vi "TDMSVisuSimple.vi"(4 "entrée d'erreur":errorcluster caption="entrée d'erreur (pas d'erreur)", 7 "chemin du fichier":path) -> (0 "sortie d'erreur":errorcluster)   [LabVIEW 2017]
panel:
  out "FileInfo":string
  out "Chaîne":string
  in  "RemoveAll":bool
  in  "DisplayAll":bool
  in  "Quitter":bool
  out "Graphe":waveform(dbl)[](graph)
  # "File information"
  # "Data"
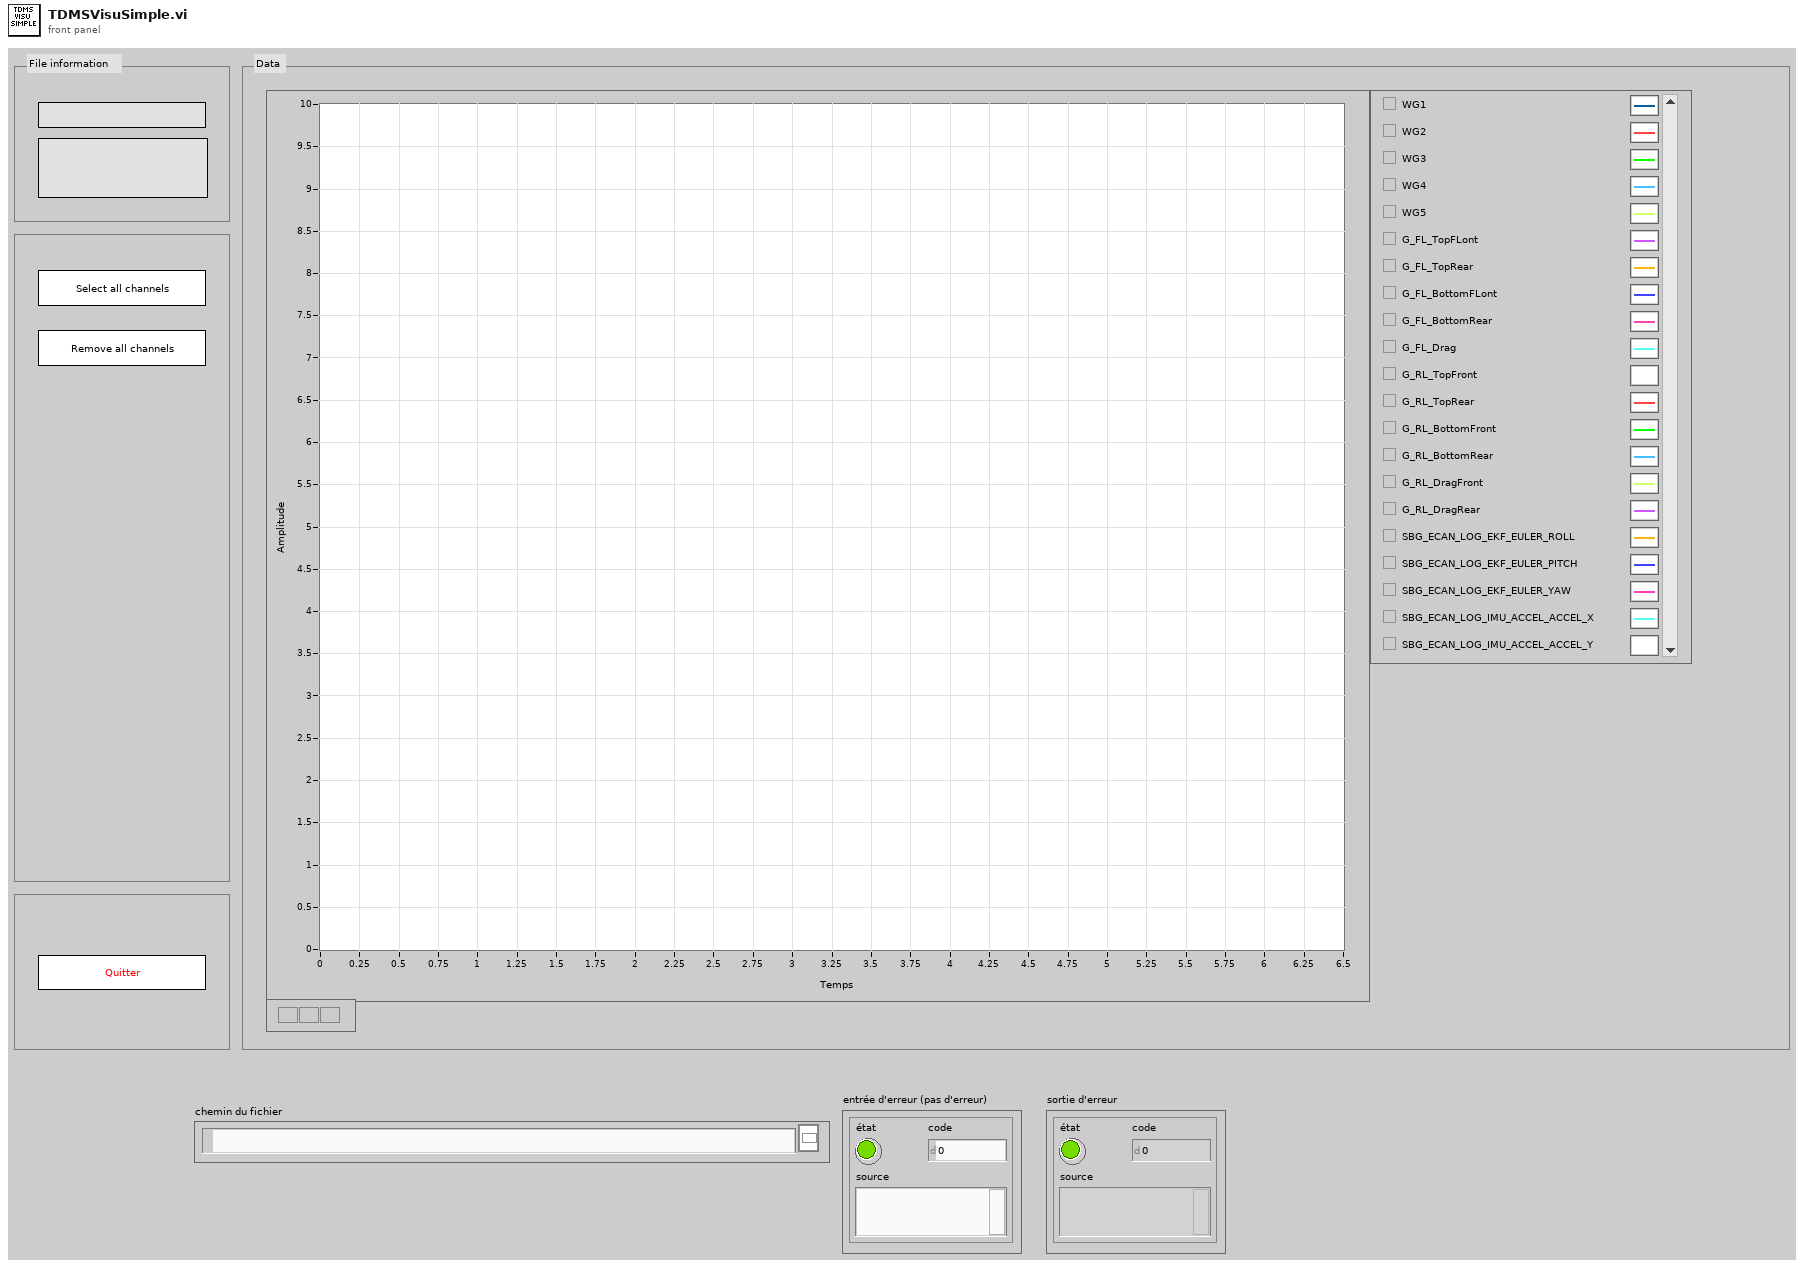
[diagram p1: front panel]
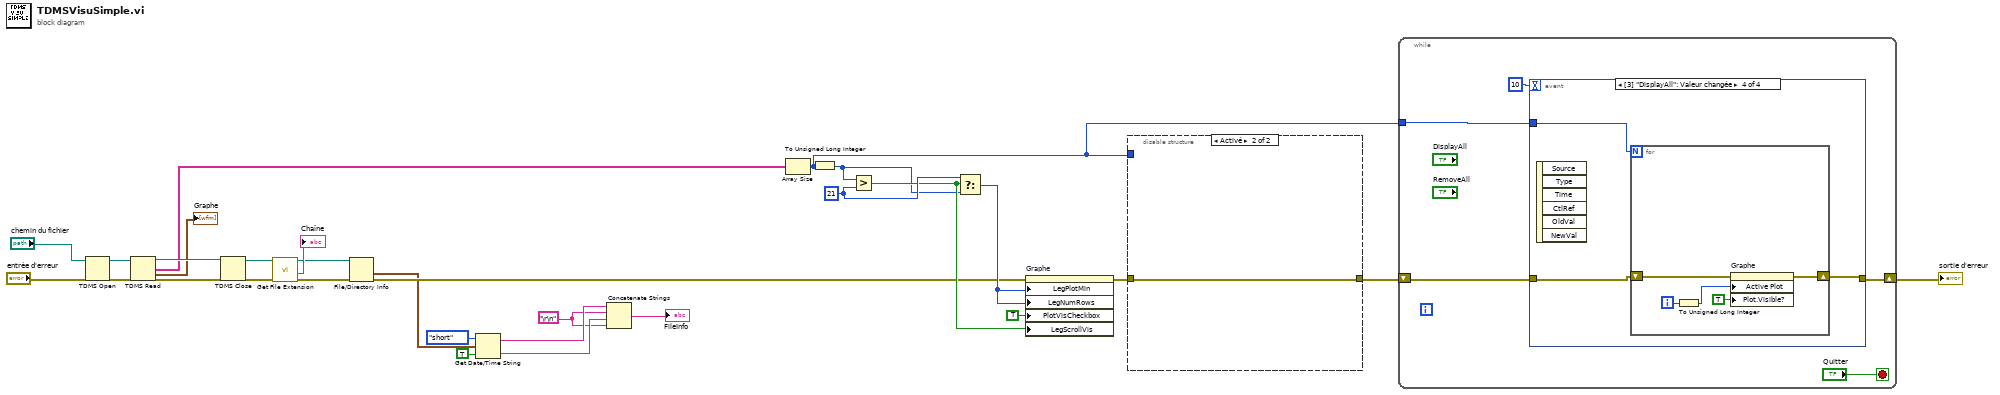
[diagram p0: block diagram]
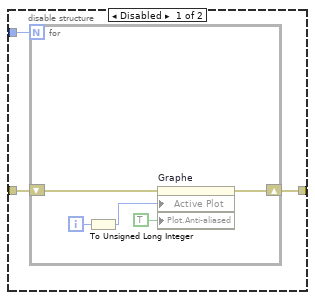
[diagram p2: hidden frame]
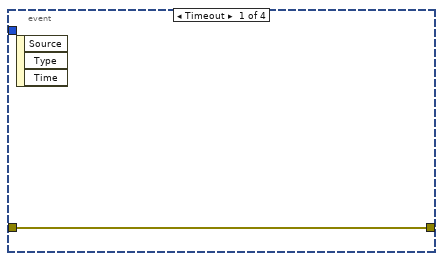
[diagram p3: hidden frame]
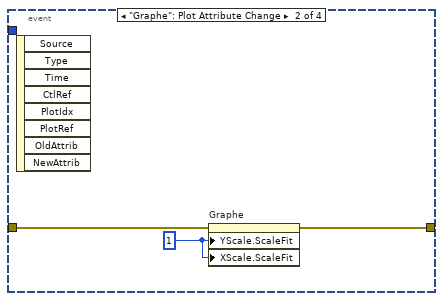
[diagram p4: hidden frame]
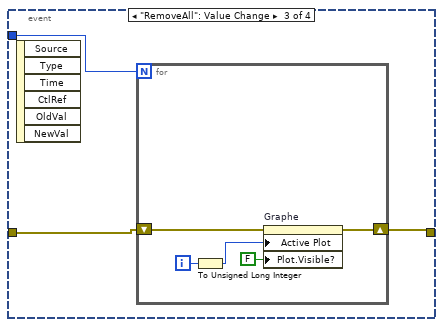
[diagram p5: hidden frame]
diagram:
  w2 = "\r\n"
  w21 = u32 21 ("y")
  n1 = TDMS Open(8:"entrée d'erreur", 11:"chemin du fichier") -> (0:w30:errorcluster, 3:w28:refnum<k34>)  [unwired: 5 in]
  n2 = TDMS Read(0:w28, 11:w30) -> (4:w27:refnum<k34>, 8:w23:string[], 10:→"Graphe":waveform(dbl)[], 15:w29:errorcluster)  [unwired: 6 in, 2 out]
  n3 = TDMS Close(8:w29, 11:w27) -> (0:w13:errorcluster, 3:w12:path)
  n4 = call <vilib>:"Get File Extension.vi"("error in (no error)"=w13, "file"=w12) -> ("error out"=w10:errorcluster, "filename without extension"=→"Chaîne":string, "dup file"=w8:path)  [unwired: 5 in, 2 out]
  n5 = File/Directory Info(path=w8, error in=w10) -> (last mod=w7:timestamp, error out=w9:errorcluster)  [unwired: 5 out]
  n6 = Get Date/Time String(date format (0)=enum16{"short", "long", "abbreviated"}."short" ("format de date (0)"), seconds (now)=w7, want seconds? (F)=TRUE ("secondes ? (F)")) -> (date string=w4:string, time string=w3:string)
  n7 = Concatenate Strings(w4, w2, w3, w2) -> (→"FileInfo":string)
  n8 = Array Size(array=w23) -> (size(s)=w14:i32)
  n9 = To Unsigned Long Integer(number=w14) -> (unsigned 32bit integer=w17:u32)
  n10 = Greater?(x=w17, y=w21) -> (0:w19:bool)
  n11 = Select(t=w21, s=w19, f=w17) -> (s? t:f=w20:u32)
  n12 = property on="Graphe" class="GraphWF (strict)"(error in=w9, "LegPlotMin"=w20, "LegNumRows"=w20, "PlotVisCheckbox"=TRUE ("Légende:Case de visibilité du tracé visible"), "LegScrollVis"=w19) -> (error out=w18:errorcluster)  [unwired: 1 in, 1 out]
  n13 = disable-structure shown="Activé" {
    disable-tunnel: w18 -> [w33 w39]
    disable-tunnel: [w32 w39] -> w16
    disable-tunnel: w14 -> [w31 _]
    frame Disabled {
      n14 = for {
        N: w31 -> [_]
        shift-right: [w35] -> w32
        shift-left: w33 -> [w36]
        i -> [w38]
        n15 = To Unsigned Long Integer(number=w38) -> (unsigned 32bit integer=w37:u32)
        n16 = property on="Graphe" class="GraphWF (strict)"(error in=w36, "Active Plot"=w37, "Plot.Anti-aliased"=TRUE ("Tracé.Lissage")) -> (error out=w35:errorcluster)  [unwired: 1 in, 1 out]
      }
    }
    frame Enabled {
    }
  }
  n17 = while {
    shift-right: [w41] -> w15
    shift-left: w16 -> [w42]
    tunnel: w14 -> [w40]
    stop <- "Quitter" stop-if-true
    n18 = event shown="[3] \"DisplayAll\": Valeur changée" {
      selector: _ -> [_ _ _ _]
      dyn-events: _ -> [_ _ _ _]
      timeout: 10 -> [_ _ _ _]
      tunnel: w42 -> [w45 w47 w51 w59]
      tunnel: [w45 w46 w49 w57] -> w41
      tunnel: w40 -> [_ _ w50 w58]
      event Timeout {
        n19 = event-data() -> ()  [unwired: 1 in, 3 out]
      }
      event "Graphe": Plot Attribute Change {
        w48 = u8 1 ("Échelle des Y.Ajuster l'échelle")
        n20 = event-data() -> ()  [unwired: 1 in, 8 out]
        n21 = property on="Graphe" class="GraphWF (strict)"(error in=w47, "YScale.ScaleFit"=w48, "XScale.ScaleFit"=w48) -> (error out=w46:errorcluster)  [unwired: 1 in, 1 out]
      }
      event "RemoveAll": Value Change {
        n22 = event-data() -> ()  [unwired: 1 in, 6 out]
        n23 = for {
          N: w50 -> [_]
          shift-right: [w53] -> w49
          shift-left: w51 -> [w54]
          i -> [w56]
          n24 = To Unsigned Long Integer(number=w56) -> (unsigned 32bit integer=w55:u32)
          n25 = property on="Graphe" class="GraphWF (strict)"(error in=w54, "Active Plot"=w55, "Plot.Visible?"=FALSE ("Tracé.Lissage")) -> (error out=w53:errorcluster)  [unwired: 1 in, 1 out]
        }
      }
      event "DisplayAll": Value Change {
        n26 = event-data() -> ()  [unwired: 1 in, 6 out]
        n27 = for {
          N: w58 -> [_]
          shift-right: [w61] -> w57
          shift-left: w59 -> [w62]
          i -> [w64]
          n28 = To Unsigned Long Integer(number=w64) -> (unsigned 32bit integer=w63:u32)
          n29 = property on="Graphe" class="GraphWF (strict)"(error in=w62, "Active Plot"=w63, "Plot.Visible?"=TRUE ("Tracé.Lissage")) -> (error out=w61:errorcluster)  [unwired: 1 in, 1 out]
        }
      }
    }
  }
  "sortie d'erreur" <- w15
